vi "read and graph co2 levels.vi"() -> ()   [LabVIEW 2013]
panel:
  out "Waveform Chart":cluster{"[0]":dbl, "[1]":dbl}(graph)
  out "read error":bool
  out "reading":dbl
  out "co2 fast":string
  in  "inter-read time (ms)":u32=250
  in  "CO2 meter serial port(s)":refnum<visa-resource-name>[](array[refnum])=["COM4"]
  in  "stop":bool
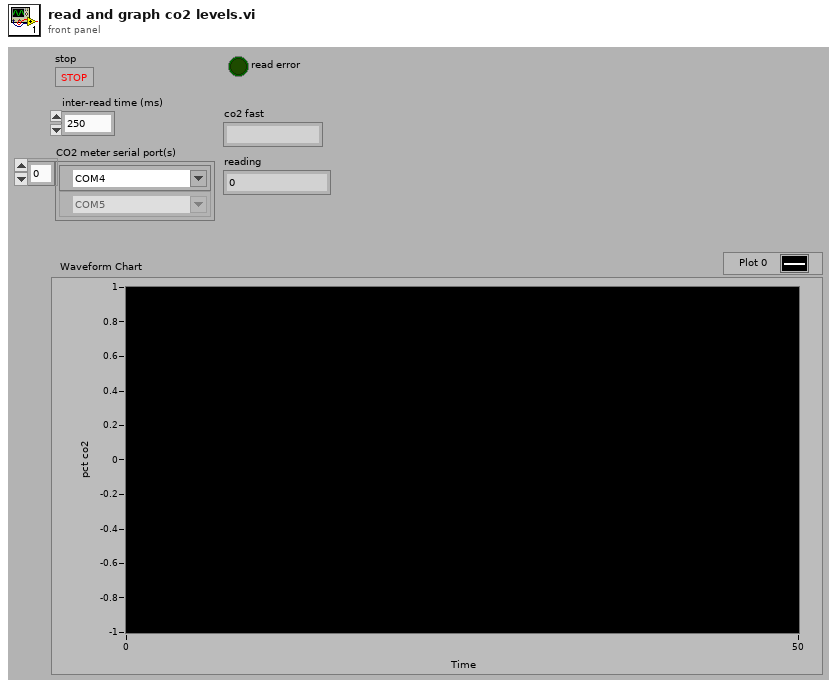
[diagram p1: front panel]
types:
  T1 = enum16{"Reset Table", "Get Values", "Add Value", "Get Table", "Get Spreadsheet"}
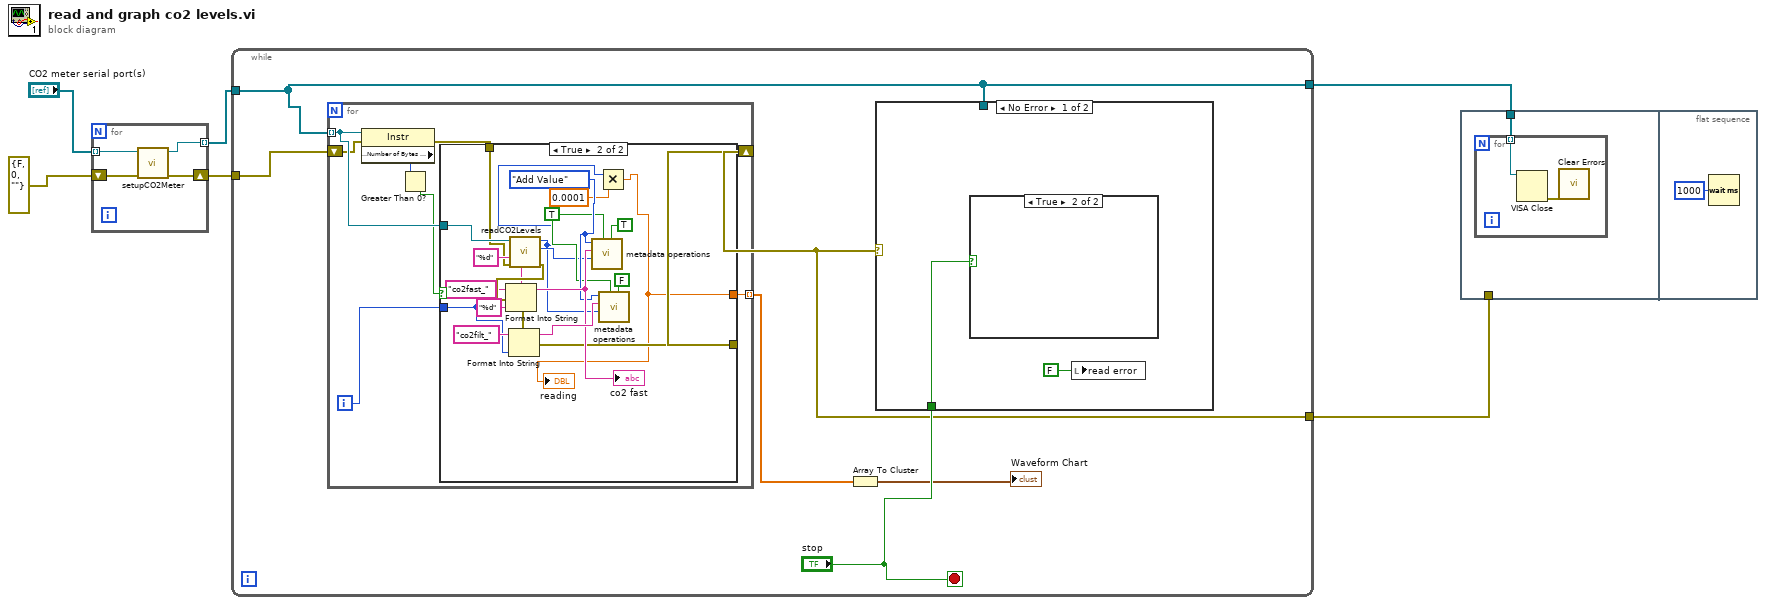
[diagram p0: block diagram]
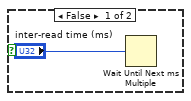
[diagram p2: hidden frame]
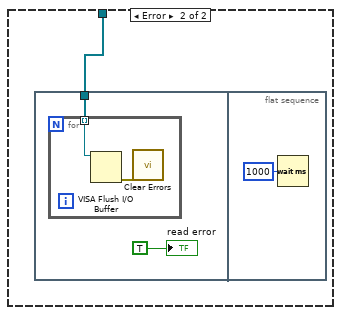
[diagram p3: hidden frame]
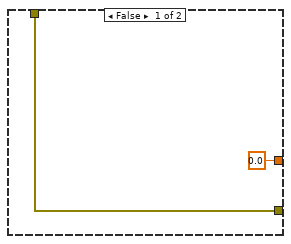
[diagram p4: hidden frame]
diagram:
  n1 = for {
    tunnel: "CO2 meter serial port(s)" -> [w9] mode=indexing
    tunnel: [w8] -> w4 mode=indexing
    shift-right: [w7] -> w3
    shift-left: errorcluster {"status"=FALSE, "code"=0, "source"=""} ("error IO") -> [w10]
    n2 = call "setupCO2Meter.vi"("VISA resource name"=w9, "error in (no error)"=w10) -> ("VISA resource name out"=w8:refnum<visa-resource-name>, "error out"=w7:errorcluster)  [unwired: 7 in]
  }
  n3 = while {
    tunnel: w4 -> [w12]
    tunnel: w3 -> [w16]
    tunnel: [w12] -> w2
    tunnel: [w11] -> w1
    stop <- "stop" stop-if-true
    n4 = for {
      tunnel: w12 -> [w32] mode=indexing
      shift-right: [w29] -> w11
      shift-left: w16 -> [w27]
      tunnel: [w26] -> w14 mode=indexing
      i -> [w31]
      n5 = property class="Instr"(reference=w32, error in=w27) -> (error out=w30:errorcluster, "Serial Settings:Number of Bytes at Serial Port"=w33:u32)  [unwired: 1 out]
      n6 = Greater Than 0?(x=w33) -> (x > 0?=w28:bool)
      n7 = case shown="True" w28 {
        tunnel: w32 -> [_ w45]
        tunnel: w31 -> [_ w44]
        tunnel: w30 -> [w35 w43]
        tunnel: [w35 w42] -> w29
        tunnel: [0.0 w36] -> w26
        frame False {
        }
        frame True {
          w40 = TRUE ("add to stackreader")
          w41 = T1."Add Value" ("Operation")
          n8 = call "readCO2Levels.vi"("error in (no error)"=w43, "VISA resource name"=w45) -> ("error IO"=w48:errorcluster, "Fast Level"=w39:i32, "Filtered Level"=w37:i32)  [unwired: 7 in]
          n9 = Format Into String(format string="%d", initial string="co2fast_", error in=w48, w44) -> (resulting string=w52:string, error out=w51:errorcluster)
          "co2 fast" <- w52
          n10 = Format Into String(format string="%d", initial string="co2filt_", error in=w51, w44) -> (resulting string=w53:string, error out=w42:errorcluster)
          n11 = call "metadata operations.vi"("add time?"=TRUE, "add to stack writer"=w40, "value"=w39, "key"=w52, "Operation"=w41) -> ()  [unwired: 3 in, 4 out]
          n12 = Multiply(x=w37, y=0.0001) -> (x*y=w36:dbl)
          "reading" <- w36
          n13 = call "metadata operations.vi"("add time?"=FALSE, "add to stack writer"=w40, "value"=w37, "key"=w53, "Operation"=w41) -> ()  [unwired: 3 in, 4 out]
        }
      }
    }
    n14 = Array To Cluster(array=w14) -> (cluster=→"Waveform Chart":cluster{"[0]":dbl, "[1]":dbl})
    n15 = case shown="No Error" w11 {
      tunnel: w12 -> [_ w20]
      tunnel: "stop" -> [w18 _]
      frame No Error {
        n16 = case shown="True" w18 {
          frame False {
            n17 = Wait Until Next ms Multiple(millisecond multiple="inter-read time (ms)") -> ()  [unwired: 1 out]
          }
          frame True {
          }
        }
        n18 = local write "read error"(FALSE ("read error")) -> ()
      }
      frame Error {
        n19 = flat-sequence {
          tunnel: w20 -> [w22]
          frame #0 {
            n20 = for {
              tunnel: w22 -> [w24] mode=indexing
              n21 = VISA Flush I/O Buffer(VISA resource name=w24) -> (error out=w23:errorcluster)  [unwired: 2 in, 1 out]
              n22 = call <vilib>:"Clear Errors.vi"("error in (no error)"=w23) -> ()  [unwired: 6 in, 1 out]
            }
            "read error" <- TRUE ("read error")
          }
          frame #1 {
            n23 = Wait (ms)(milliseconds to wait=u32 1000) -> ()  [unwired: 1 out]
          }
        }
      }
    }
  }
  n24 = flat-sequence {
    tunnel: w2 -> [w56]
    tunnel: w1 -> [_]
    frame #0 {
      n25 = for {
        tunnel: w56 -> [w58] mode=indexing
        n26 = VISA Close(VISA resource name=w58) -> (error out=w57:errorcluster)  [unwired: 1 in]
        n27 = call <vilib>:"Clear Errors.vi"("error in (no error)"=w57) -> ()  [unwired: 6 in, 1 out]
      }
    }
    frame #1 {
      n28 = Wait (ms)(milliseconds to wait=u32 1000) -> ()  [unwired: 1 out]
    }
  }
